vi "ManualClimb.vi"   [LabVIEW 2020]
uses:
  Robot Global Data.vi
  Swerve Global Variables.vi
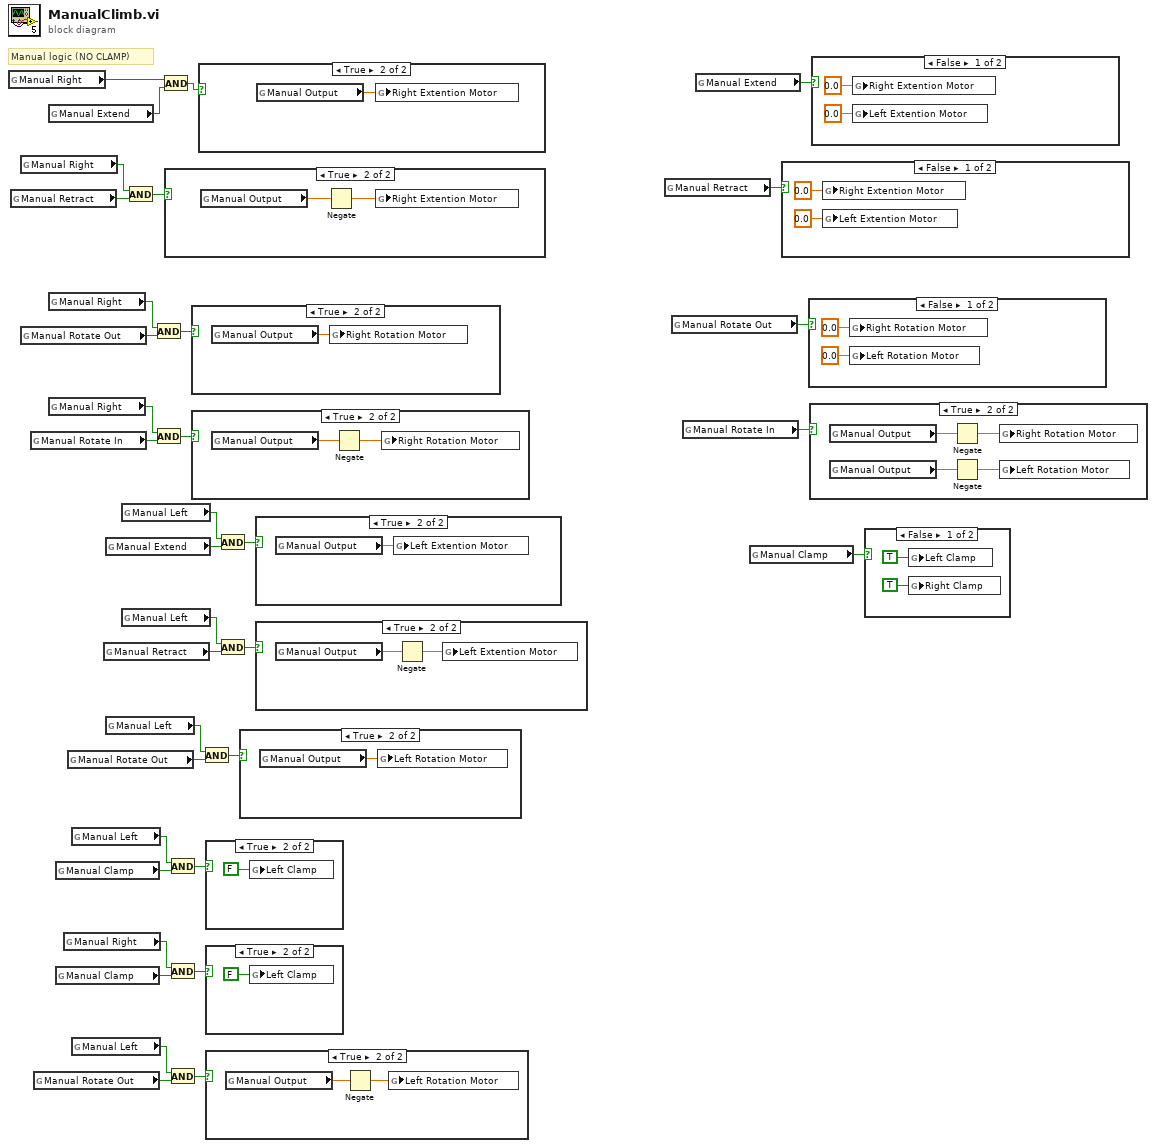
[diagram p0: block diagram]
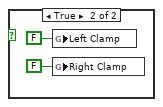
[diagram p2: hidden frame]
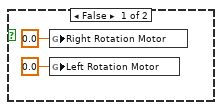
[diagram p3: hidden frame]
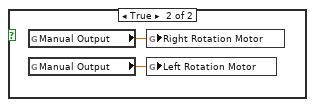
[diagram p4: hidden frame]
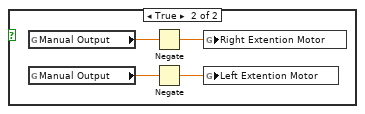
[diagram p5: hidden frame]
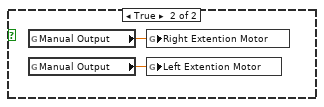
[diagram p6: hidden frame]
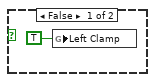
[diagram p7: hidden frame]
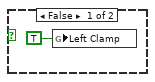
[diagram p8: hidden frame]
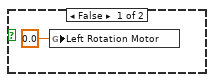
[diagram p9: hidden frame]
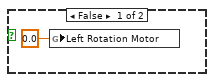
[diagram p10: hidden frame]
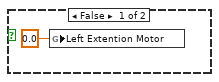
[diagram p11: hidden frame]
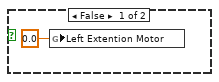
[diagram p12: hidden frame]
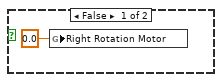
[diagram p13: hidden frame]
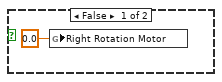
[diagram p14: hidden frame]
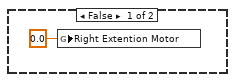
[diagram p15: hidden frame]
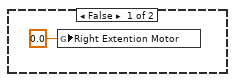
[diagram p16: hidden frame]
diagram:
  # "Manual logic (NO CLAMP)"
  n1 = global read "Robot Global Data.vi" "Manual Right"() -> (w7:bool)
  n2 = global read "Robot Global Data.vi" "Manual Retract"() -> (w10:bool)
  n3 = global read "Robot Global Data.vi" "Manual Right"() -> (w9:bool)
  n4 = global read "Robot Global Data.vi" "Manual Rotate Out"() -> (w14:bool)
  n5 = global read "Robot Global Data.vi" "Manual Rotate In"() -> (w17:bool)
  n6 = global read "Robot Global Data.vi" "Manual Rotate Out"() -> (w29:bool)
  n7 = global read "Robot Global Data.vi" "Manual Extend"() -> (w6:bool)
  n8 = global read "Robot Global Data.vi" "Manual Right"() -> (w13:bool)
  n9 = global read "Robot Global Data.vi" "Manual Right"() -> (w16:bool)
  n10 = global read "Robot Global Data.vi" "Manual Clamp"() -> (w31:bool)
  n11 = global read "Robot Global Data.vi" "Manual Clamp"() -> (w33:bool)
  n12 = global read "Robot Global Data.vi" "Manual Right"() -> (w32:bool)
  n13 = global read "Robot Global Data.vi" "Manual Rotate Out"() -> (w26:bool)
  n14 = global read "Robot Global Data.vi" "Manual Left"() -> (w30:bool)
  n15 = global read "Robot Global Data.vi" "Manual Left"() -> (w28:bool)
  n16 = global read "Robot Global Data.vi" "Manual Retract"() -> (w22:bool)
  n17 = global read "Robot Global Data.vi" "Manual Extend"() -> (w18:bool)
  n18 = global read "Robot Global Data.vi" "Manual Left"() -> (w25:bool)
  n19 = global read "Robot Global Data.vi" "Manual Left"() -> (w19:bool)
  n20 = global read "Robot Global Data.vi" "Manual Left"() -> (w21:bool)
  n21 = And(x=w9, y=w10) -> (x .and. y?=w11:bool)
  n22 = And(x=w13, y=w14) -> (x .and. y?=w12:bool)
  n23 = And(x=w16, y=w17) -> (x .and. y?=w15:bool)
  n24 = And(x=w7, y=w6) -> (x .and. y?=w8:bool)
  n25 = case shown="True" w11 {
    frame False {
      n26 = global write "Swerve Global Variables.vi" "Right Extention Motor"(0.0 ("Right Rotation Motor")) -> ()
    }
    frame True {
      n27 = global read "Swerve Global Variables.vi" "Manual Output"() -> (w38:dbl)
      n28 = Negate(x=w38) -> (-x=w37:dbl)
      n29 = global write "Swerve Global Variables.vi" "Right Extention Motor"(w37) -> ()
    }
  }
  n30 = And(x=w30, y=w31) -> (x .and. y?=w35:bool)
  n31 = And(x=w32, y=w33) -> (x .and. y?=w34:bool)
  n32 = And(x=w28, y=w29) -> (x .and. y?=w27:bool)
  n33 = case shown="True" w12 {
    frame False {
      n34 = global write "Swerve Global Variables.vi" "Right Rotation Motor"(0.0 ("Right Extention Motor")) -> ()
    }
    frame True {
      n35 = global read "Swerve Global Variables.vi" "Manual Output"() -> (w40:dbl)
      n36 = global write "Swerve Global Variables.vi" "Right Rotation Motor"(w40) -> ()
    }
  }
  n37 = case shown="True" w15 {
    frame False {
      n38 = global write "Swerve Global Variables.vi" "Right Rotation Motor"(0.0 ("Right Extention Motor")) -> ()
    }
    frame True {
      n39 = global read "Swerve Global Variables.vi" "Manual Output"() -> (w43:dbl)
      n40 = Negate(x=w43) -> (-x=w42:dbl)
      n41 = global write "Swerve Global Variables.vi" "Right Rotation Motor"(w42) -> ()
    }
  }
  n42 = case shown="True" w8 {
    frame False {
      n43 = global write "Swerve Global Variables.vi" "Right Extention Motor"(0.0 ("Right Rotation Motor")) -> ()
    }
    frame True {
      n44 = global read "Swerve Global Variables.vi" "Manual Output"() -> (w45:dbl)
      n45 = global write "Swerve Global Variables.vi" "Right Extention Motor"(w45) -> ()
    }
  }
  n46 = And(x=w25, y=w26) -> (x .and. y?=w24:bool)
  n47 = case shown="True" w35 {
    frame False {
      n48 = global write "Robot Global Data.vi" "Left Clamp"(TRUE ("Left Clamp")) -> ()
    }
    frame True {
      n49 = global write "Robot Global Data.vi" "Left Clamp"(FALSE ("Left Clamp")) -> ()
    }
  }
  n50 = case shown="True" w34 {
    frame False {
      n51 = global write "Robot Global Data.vi" "Left Clamp"(TRUE ("Left Clamp")) -> ()
    }
    frame True {
      n52 = global write "Robot Global Data.vi" "Left Clamp"(FALSE ("Left Clamp")) -> ()
    }
  }
  n53 = case shown="True" w27 {
    frame False {
      n54 = global write "Swerve Global Variables.vi" "Left Rotation Motor"(0.0 ("Left Rotation Motor")) -> ()
    }
    frame True {
      n55 = global read "Swerve Global Variables.vi" "Manual Output"() -> (w51:dbl)
      n56 = Negate(x=w51) -> (-x=w52:dbl)
      n57 = global write "Swerve Global Variables.vi" "Left Rotation Motor"(w52) -> ()
    }
  }
  n58 = And(x=w19, y=w18) -> (x .and. y?=w20:bool)
  n59 = And(x=w21, y=w22) -> (x .and. y?=w23:bool)
  n60 = case shown="True" w24 {
    frame False {
      n61 = global write "Swerve Global Variables.vi" "Left Rotation Motor"(0.0 ("Left Rotation Motor")) -> ()
    }
    frame True {
      n62 = global read "Swerve Global Variables.vi" "Manual Output"() -> (w54:dbl)
      n63 = global write "Swerve Global Variables.vi" "Left Rotation Motor"(w54) -> ()
    }
  }
  n64 = case shown="True" w20 {
    frame False {
      n65 = global write "Swerve Global Variables.vi" "Left Extention Motor"(0.0 ("Left Extention Motor")) -> ()
    }
    frame True {
      n66 = global read "Swerve Global Variables.vi" "Manual Output"() -> (w56:dbl)
      n67 = global write "Swerve Global Variables.vi" "Left Extention Motor"(w56) -> ()
    }
  }
  n68 = case shown="True" w23 {
    frame False {
      n69 = global write "Swerve Global Variables.vi" "Left Extention Motor"(0.0 ("Left Extention Motor")) -> ()
    }
    frame True {
      n70 = global read "Swerve Global Variables.vi" "Manual Output"() -> (w59:dbl)
      n71 = Negate(x=w59) -> (-x=w58:dbl)
      n72 = global write "Swerve Global Variables.vi" "Left Extention Motor"(w58) -> ()
    }
  }
  n73 = global read "Robot Global Data.vi" "Manual Retract"() -> (w4:bool)
  n74 = global read "Robot Global Data.vi" "Manual Rotate Out"() -> (w3:bool)
  n75 = global read "Robot Global Data.vi" "Manual Rotate In"() -> (w2:bool)
  n76 = global read "Robot Global Data.vi" "Manual Extend"() -> (w5:bool)
  n77 = global read "Robot Global Data.vi" "Manual Clamp"() -> (w1:bool)
  n78 = case shown="False" w4 {
    frame False {
      n79 = global write "Swerve Global Variables.vi" "Right Extention Motor"(0.0 ("Right Rotation Motor")) -> ()
      n80 = global write "Swerve Global Variables.vi" "Left Extention Motor"(0.0 ("Right Rotation Motor")) -> ()
    }
    frame True {
      n81 = global read "Swerve Global Variables.vi" "Manual Output"() -> (w65:dbl)
      n82 = global read "Swerve Global Variables.vi" "Manual Output"() -> (w63:dbl)
      n83 = Negate(x=w65) -> (-x=w64:dbl)
      n84 = Negate(x=w63) -> (-x=w62:dbl)
      n85 = global write "Swerve Global Variables.vi" "Right Extention Motor"(w64) -> ()
      n86 = global write "Swerve Global Variables.vi" "Left Extention Motor"(w62) -> ()
    }
  }
  n87 = case shown="False" w3 {
    frame False {
      n88 = global write "Swerve Global Variables.vi" "Right Rotation Motor"(0.0 ("Right Extention Motor")) -> ()
      n89 = global write "Swerve Global Variables.vi" "Left Rotation Motor"(0.0 ("Right Extention Motor")) -> ()
    }
    frame True {
      n90 = global read "Swerve Global Variables.vi" "Manual Output"() -> (w69:dbl)
      n91 = global read "Swerve Global Variables.vi" "Manual Output"() -> (w68:dbl)
      n92 = global write "Swerve Global Variables.vi" "Right Rotation Motor"(w69) -> ()
      n93 = global write "Swerve Global Variables.vi" "Left Rotation Motor"(w68) -> ()
    }
  }
  n94 = case shown="True" w2 {
    frame False {
      n95 = global write "Swerve Global Variables.vi" "Right Rotation Motor"(0.0 ("Right Extention Motor")) -> ()
      n96 = global write "Swerve Global Variables.vi" "Left Rotation Motor"(0.0 ("Right Extention Motor")) -> ()
    }
    frame True {
      n97 = global read "Swerve Global Variables.vi" "Manual Output"() -> (w75:dbl)
      n98 = global read "Swerve Global Variables.vi" "Manual Output"() -> (w73:dbl)
      n99 = Negate(x=w75) -> (-x=w74:dbl)
      n100 = Negate(x=w73) -> (-x=w72:dbl)
      n101 = global write "Swerve Global Variables.vi" "Right Rotation Motor"(w74) -> ()
      n102 = global write "Swerve Global Variables.vi" "Left Rotation Motor"(w72) -> ()
    }
  }
  n103 = case shown="False" w5 {
    frame False {
      n104 = global write "Swerve Global Variables.vi" "Right Extention Motor"(0.0 ("Right Rotation Motor")) -> ()
      n105 = global write "Swerve Global Variables.vi" "Left Extention Motor"(0.0 ("Right Rotation Motor")) -> ()
    }
    frame True {
      n106 = global read "Swerve Global Variables.vi" "Manual Output"() -> (w79:dbl)
      n107 = global read "Swerve Global Variables.vi" "Manual Output"() -> (w78:dbl)
      n108 = global write "Swerve Global Variables.vi" "Right Extention Motor"(w79) -> ()
      n109 = global write "Swerve Global Variables.vi" "Left Extention Motor"(w78) -> ()
    }
  }
  n110 = case shown="False" w1 {
    frame False {
      n111 = global write "Robot Global Data.vi" "Left Clamp"(TRUE ("Left Clamp")) -> ()
      n112 = global write "Robot Global Data.vi" "Right Clamp"(TRUE ("Left Clamp")) -> ()
    }
    frame True {
      n113 = global write "Robot Global Data.vi" "Left Clamp"(FALSE ("Left Clamp")) -> ()
      n114 = global write "Robot Global Data.vi" "Right Clamp"(FALSE ("Left Clamp")) -> ()
    }
  }
